vi "enqueue_pressure_auto_offset.vi"(0 "autoOffsetPsatQueue":refnum<queue>, 1 "# to average":dbl=100.0 format="%#_13g", 2 "Auto Offset":refnum<vi>, 3 "Pressure/Temperature/Mixture Properties":T1={"Line Densities\n[g/cm^3]"={"Vapor Line"=0.15445189986836314, "Liquid Line"=0.25755261741892205}, "Mixture Properties"={"Enthalpy"=195841526251804.2, "Quality [-]"=-10.825375459319764}, "[Readings]"={"Streamwise P"=-3074.4228785963764, "Streamwise T"=nan, "Streamwise Sat P"=nan, "Streamwise Sat T"=nan, "Liquid Tank P"=3834985507386.06, "Liquid Tank T"=456.4106234658312, "Liquid Tank Sat P"=1736233577203.0627, "Liquid Tank Sat T"=492.17973224367375, "Separator P"=179910.46497250997, "Separator T"=-13120080.345725078, "Separator Sat P"=0.0, "Separator Sat T"=30.62899308837065, "Liquid Inlet P"=185261.09355383943, "Liquid Inlet T"=508.4593419640114, "Liquid Inlet Sat P"=12378986008470.418, "Liquid Inlet Sat T"=31.430570229281372, "Vapor Tank P"=108956.35947325415, "Vapor Tank T"=-10372083.904135285, "Vapor Tank Sat P"=0.0, "Vapor Tank Sat T"=16.912041354361705, "Vapor Inlet P"=379651.1166364239, "Vapor Inlet T"=381.53210552887515, "Vapor Inlet Sat P"=102884868683.01198, "Vapor Inlet Sat T"=51.054688909951395, "Upper Test Section P"=44976.833741485905, "Upper Test Section T"=-16719245.882515587, "Upper Test Section Sat P"=0.0, "Upper Test Section Sat T"=-7.288297090299707, "Lower Test Section P"=4027555317727.7935, "Lower Test Section T"=527.5685201983387, "Lower Test Section Sat P"=25461496462993.004, "Lower Test Section Sat T"=493.51977461723476}, "Condensor/Evaporator\nTemperature"={"Bottom Evaporator\nTemperature [C]"=0.011951520540655883, "Bottom Condensor\nTemperature [C]"=-36481825.305210106, "Top Evaporator\nTemperature [C]"=-0.005944396537208351, "Top Condensor\nTemperature [C]"=-0.03695927054192248}, "Test Section \nPressure [Pa]"=62496.106498599445, "Heater Temperatures [C]"={"Vapor Tank"=0.025136174921612436, "Liquid Tank"=0.021290742477967885}}, 4 "Auto Offset ProgressBar":refnum<vi>) -> ()   [LabVIEW 2015]
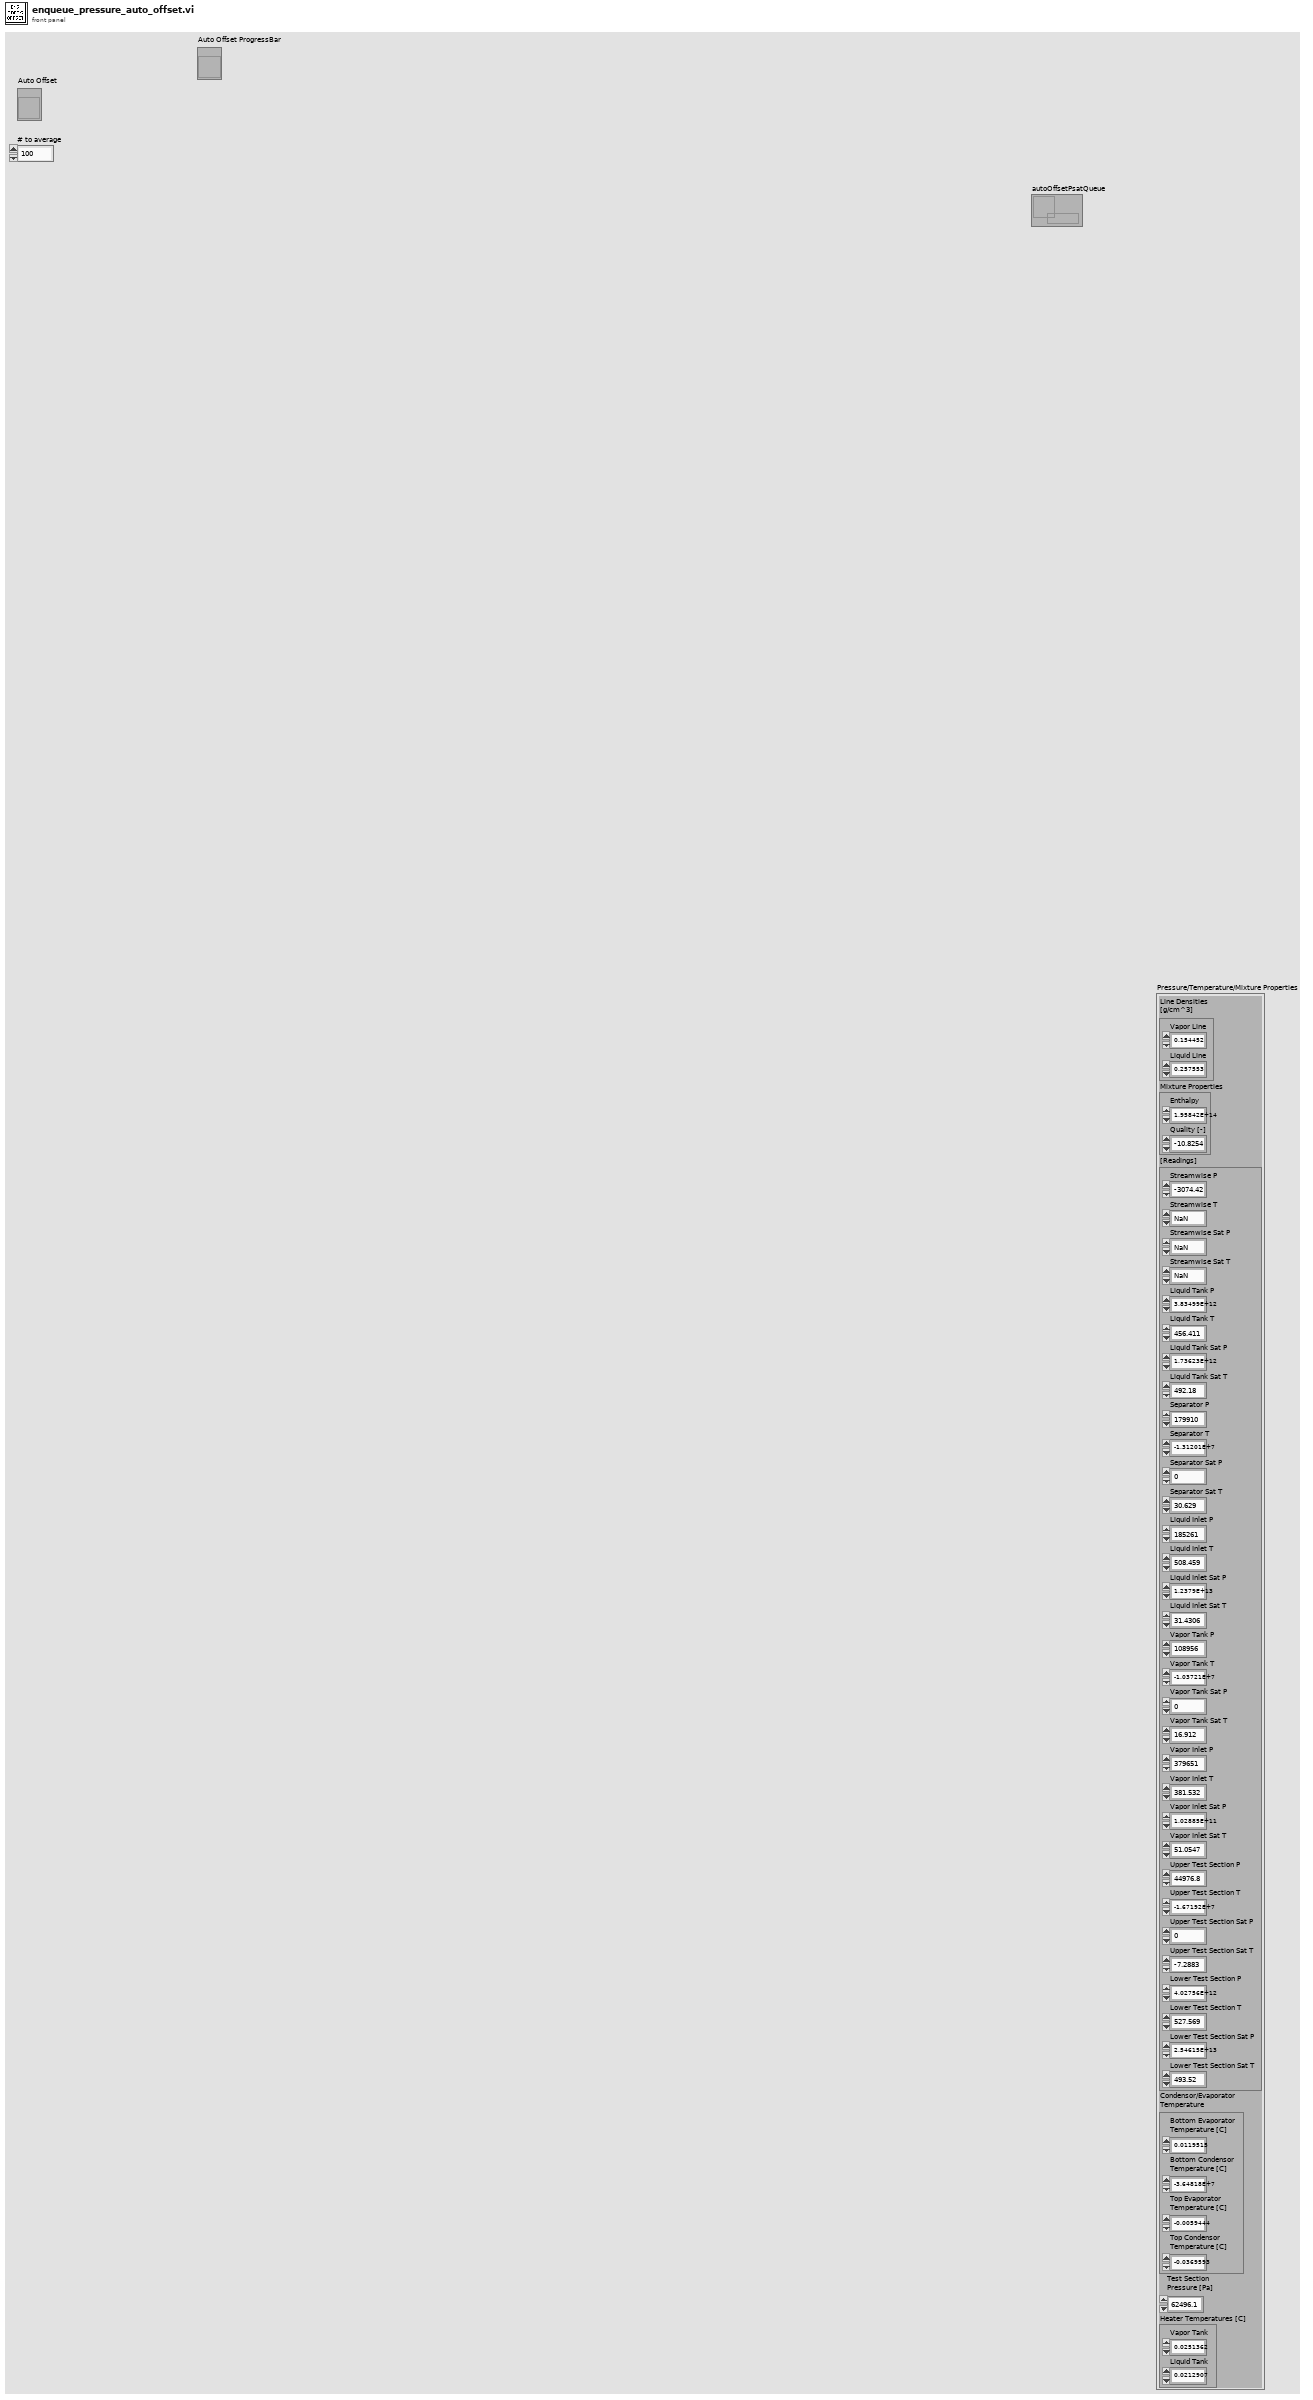
[diagram p1: front panel]
types:
  T1 = cluster{"Line Densities\n[g/cm^3]":cluster{"Vapor Line":dbl, "Liquid Line":dbl}, "Mixture Properties":cluster{"Enthalpy":dbl, "Quality [-]":dbl}, "[Readings]":cluster{"Streamwise P":dbl, "Streamwise T":dbl, "Streamwise Sat P":dbl, "Streamwise Sat T":dbl, "Liquid Tank P":dbl, "Liquid Tank T":dbl, "Liquid Tank Sat P":dbl, "Liquid Tank Sat T":dbl, "Separator P":dbl, "Separator T":dbl, "Separator Sat P":dbl, "Separator Sat T":dbl, "Liquid Inlet P":dbl, "Liquid Inlet T":dbl, "Liquid Inlet Sat P":dbl, "Liquid Inlet Sat T":dbl, "Vapor Tank P":dbl, "Vapor Tank T":dbl, "Vapor Tank Sat P":dbl, "Vapor Tank Sat T":dbl, "Vapor Inlet P":dbl, "Vapor Inlet T":dbl, "Vapor Inlet Sat P":dbl, "Vapor Inlet Sat T":dbl, "Upper Test Section P":dbl, "Upper Test Section T":dbl, "Upper Test Section Sat P":dbl, "Upper Test Section Sat T":dbl, "Lower Test Section P":dbl, "Lower Test Section T":dbl, "Lower Test Section Sat P":dbl, "Lower Test Section Sat T":dbl}, "Condensor/Evaporator\nTemperature":cluster{"Bottom Evaporator\nTemperature [C]":dbl, "Bottom Condensor\nTemperature [C]":dbl, "Top Evaporator\nTemperature [C]":dbl, "Top Condensor\nTemperature [C]":dbl}, "Test Section \nPressure [Pa]":dbl, "Heater Temperatures [C]":cluster{"Vapor Tank":dbl, "Liquid Tank":dbl}}
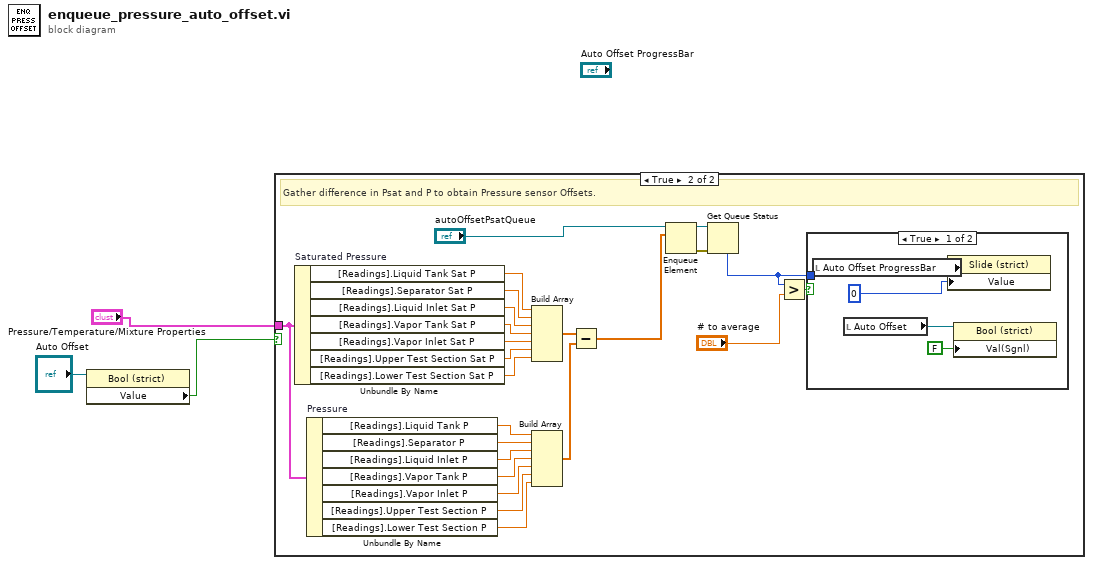
[diagram p0: block diagram]
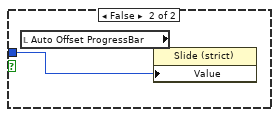
[diagram p3: hidden frame]
diagram:
  n1 = property class="Bool (strict)"(reference="Auto Offset") -> ("Value"=w1:bool)  [unwired: 1 in, 2 out]
  n2 = case shown="True" w1 {
    tunnel: "Pressure/Temperature/Mixture Properties" -> [_ w5]
    frame False {
    }
    frame True {
      # "Gather difference in Psat and P to obtain Pressure sensor Offsets."
      n3 = Unbundle By Name "Saturated Pressure"(w5) -> ("[Readings].Liquid Tank Sat P"=w12:dbl, "[Readings].Separator Sat P"=w13:dbl, "[Readings].Liquid Inlet Sat P"=w14:dbl, "[Readings].Vapor Tank Sat P"=w15:dbl, "[Readings].Vapor Inlet Sat P"=w16:dbl, "[Readings].Upper Test Section Sat P"=w17:dbl, "[Readings].Lower Test Section Sat P"=w18:dbl)
      n4 = Unbundle By Name "Pressure"(w5) -> ("[Readings].Liquid Tank P"=w27:dbl, "[Readings].Separator P"=w26:dbl, "[Readings].Liquid Inlet P"=w25:dbl, "[Readings].Vapor Tank P"=w24:dbl, "[Readings].Vapor Inlet P"=w23:dbl, "[Readings].Upper Test Section P"=w22:dbl, "[Readings].Lower Test Section P"=w21:dbl)
      n5 = Build Array(w12, w13, w14, w15, w16, w17, w18) -> (w10:dbl[])
      n6 = Build Array(w27, w26, w25, w24, w23, w22, w21) -> (w9:dbl[])
      n7 = Subtract(x=w10, y=w9) -> (x-y=w11:dbl[])
      n8 = Enqueue Element(queue="autoOffsetPsatQueue", element=w11) -> (queue out=w20:refnum<queue>, error out=w19:errorcluster)  [unwired: 2 in, 1 out]
      n9 = Get Queue Status(queue=w20, error in (no error)=w19) -> (# elements in queue=w6:i32)  [unwired: 1 in, 7 out]
      n10 = Greater?(x=w6, y="# to average") -> (0:w8:bool)
      n11 = case shown="True" w8 {
        tunnel: w6 -> [_ w33]
        frame True {
          n12 = local read "Auto Offset ProgressBar"() -> (w28:refnum<vi>)
          n13 = local read "Auto Offset"() -> (w30:refnum<vi>)
          n14 = property class="Slide (strict)"(reference=w28, "Value"=u32 0 ("Auto Offset Progress")) -> ()  [unwired: 1 in, 2 out]
          n15 = property class="Bool (strict)"(reference=w30, "Val(Sgnl)"=FALSE) -> ()  [unwired: 1 in, 2 out]
        }
        frame False {
          n16 = local read "Auto Offset ProgressBar"() -> (w32:refnum<vi>)
          n17 = property class="Slide (strict)"(reference=w32, "Value"=w33) -> ()  [unwired: 1 in, 2 out]
        }
      }
    }
  }
